vi "Close Config.vi"(8 "error in (no error)":errorcluster, 11 "Configuration File In":refnum<class "Mock Configuration.lvclass">) -> (0 "error out":errorcluster, 3 "Configuration File Out":refnum<class "Mock Configuration.lvclass">)   [LabVIEW 2020, in "Mock Configuration.lvclass"]
doc: "High-level function for opening configuration file data from Process class."
uses:
  Mock Configuration.lvclass
  C:/Program Files (x86)/National Instruments/LabVIEW 2020/vi.lib/Astemes/LMock/Mock.lvclass
  <vilib>/Astemes/LMock/Mock.lvclass
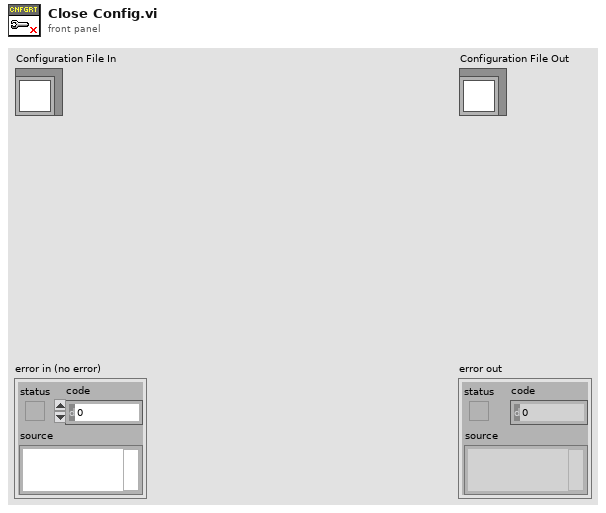
[diagram p1: front panel]
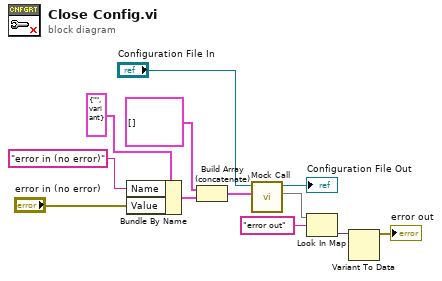
[diagram p0: block diagram]
diagram:
  n1 = Bundle By Name(cluster=cluster{"Name":string, "Value":variant} {"Name"="", "Value"=variant} ("element"), "Name"="error in (no error)", "Value"="error in (no error)") -> (w1:cluster{"Name":string, "Value":variant})
  n2 = Build Array (concatenate)(cluster{"Name":string, "Value":variant}[] [] ("Control Values"), w1) -> (w9:cluster{"Name":string, "Value":variant}[])
  n3 = call <vilib>:"Mock Call.vi"("Control Values"=w9, "Mock In"="Configuration File In") -> ("Return Values"=w7:map{string, variant}, "Mock Out"=→"Configuration File Out":refnum<class "Mock Configuration.lvclass">)  [unwired: 8 in]
  n4 = Look In Map(map=w7, key="error out") -> (value=w5:variant)  [unwired: 1 in, 1 out]
  n5 = Variant To Data(Variant=w5) -> (data=→"error out":errorcluster)  [unwired: 2 in, 1 out]
